vi "add_uint16.vi"   [LabVIEW 2012]
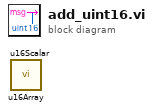
[diagram p0: block diagram]
diagram:
  n1 = call <userlib>:"u16Array.vi"() -> ()  [unwired: 5 in, 1 out]
  n2 = call <userlib>:"u16Scalar.vi"() -> ()  [unwired: 5 in, 1 out]
